vi "configGrab.vi"(8 "error in (no error)":errorcluster, 9 "Number of Buffers":u32=3, 10 "Continuous?":T1=enum."Continuous", 11 "camera in":refnum<class "camera.lvclass">) -> (0 "error out":errorcluster, 3 "camera out":refnum<class "camera.lvclass">)   [LabVIEW 2017, in "camera.lvclass"]
uses:
  camera.lvclass
  <vilib>/vision/driver/IMAQdx.llb/IMAQdx Acquisition Mode.ctl
  <vilib>/vision/driver/NI_Vision_Acquisition_Software.lvlib
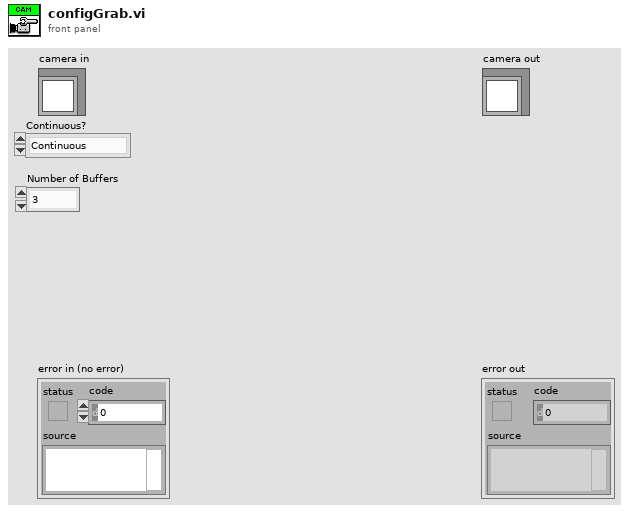
[diagram p1: front panel]
types:
  T1 = typedef "NI_Vision_Acquisition_Software.lvlib/IMAQdx Acquisition Mode.ctl" = enum32{"One Shot", "Continuous"}
  T2 = typedef "IMAQdx.ctl" = refnum<k21>
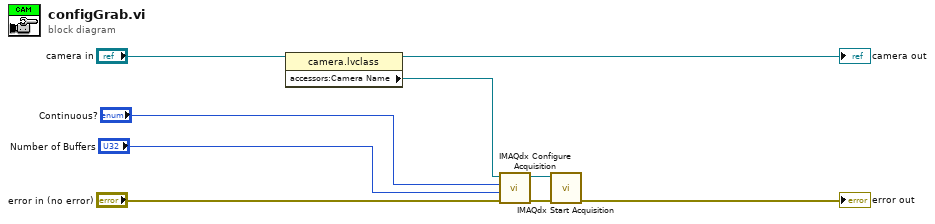
[diagram p0: block diagram]
diagram:
  n1 = property class="camera.lvclass"(reference="camera in") -> (reference out=→"camera out":refnum<class "camera.lvclass">, "accessors:Camera Name"=w3:refnum<k21>)  [unwired: 1 in, 1 out]
  n2 = call <vilib>:"IMAQdx Configure Acquisition.vi"("error in"="error in (no error)", "Number of Buffers"="Number of Buffers", "Continuous?"="Continuous?", "Session In"=w3) -> ("error out"=w8:errorcluster, "Session Out"=w9:T2)  [unwired: 6 out]
  n3 = call <vilib>:"IMAQdx Start Acquisition.vi"("error in"=w8, "Session In"=w9) -> ("error out"=→"error out":errorcluster)  [unwired: 9 out]
